vi "KalibrationRefMicro.vi"() -> ()   [LabVIEW 2012]
uses:
  <vilib>/addons/Sound and Vibration/svt_DAQmx/Configuration XControl/SVX NI-DAQmx AI Configuration XControl.xctl
  <vilib>/DAQmx/read.llb/DAQmx Read (Analog 1D Wfm NChan 1Samp).vi
  <vilib>/DAQmx/miscellaneous.llb/DAQmx Fill In Error Info.vi
panel:
  out "Waveform Graph":waveform(dbl)[](graph)
  in  "SVX NI-DAQmx AI Configuration XControl":refnum<k21>(xcontrol)
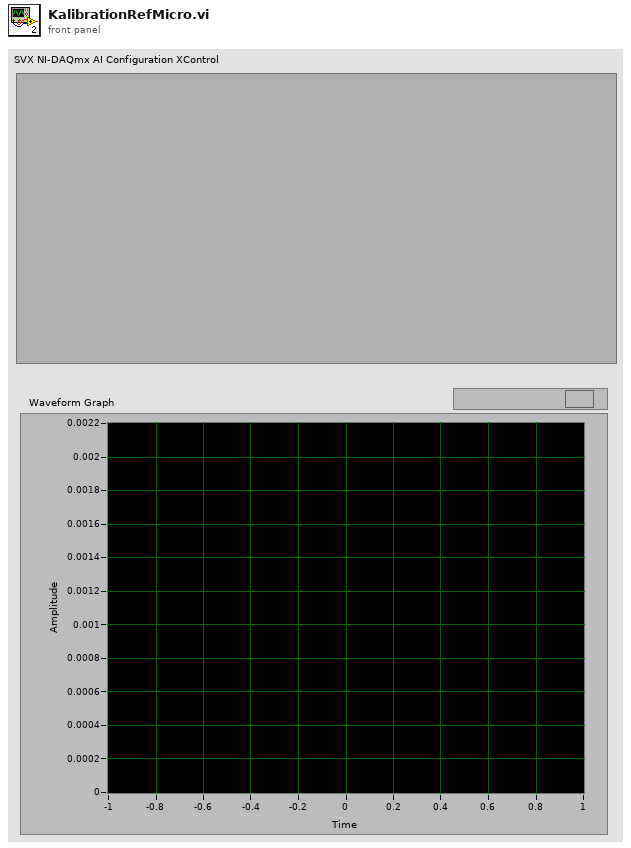
[diagram p1: front panel]
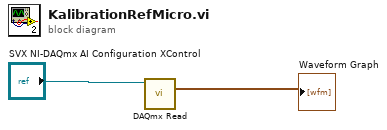
[diagram p0: block diagram]
diagram:
  n1 = call-poly <vilib>:"DAQmx Read.vi"("task/channels in"="SVX NI-DAQmx AI Configuration XControl") -> ("data"=→"Waveform Graph":waveform(dbl)[])  [unwired: 12 in, 2 out]
